vi "RT_DAQ Loop.vi"(8 "error in":errorcluster, 11 "Main Data":T1) -> (0 "error out":errorcluster)   [LabVIEW 2018]
uses:
  Data Def/RT_Main Data.ctl
  Data Def/RT_FPGA VI Reference.ctl
  Data Def/RT_Request Data.ctl
  <vilib>/Platform/TimedLoop/XDataNode/timing_clust.ctl
  <vilib>/Platform/TimedLoop/XDataNode/nitl_modes.ctl
  <vilib>/Platform/TimedLoop/XDataNode/wakeup.ctl
  Data Def/RT_Normal FGV Method.ctl
  <vilib>/Analysis/baseanly.llb/Mean (DBL).vi
  <vilib>/Utility/error.llb/Error Cluster From Error Code.vi
  <vilib>/rvi/errors/niLvFpgaAdjustHostInterfaceError.vi
  <vilib>/platform/TimedLoop/XDataNode/XDataNode.xnode
  <vilib>/rvi/interface/nirviReadWriteControl/nirviReadWriteControl.xnode
  <vilib>/Platform/TimedLoop/XDataNode/XDNodeRunTimeDep.lvlib
  NiFpgaLv.dll
  <vilib>/rvi/interface/Simulation/niFpgaSimulationCallBeginRW.vi
  <vilib>/Analysis/NI_AALBase.lvlib
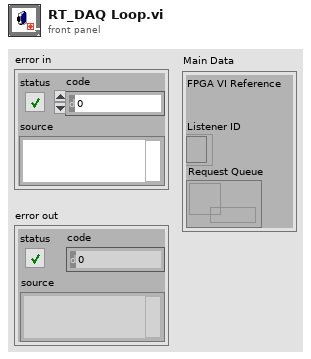
[diagram p1: front panel]
types:
  T1 = typedef "RT_Main Data.ctl" = cluster{"FPGA VI Reference":T2, "Listener ID":refnum<k5>, "Request Queue":refnum<queue>}
  T2 = typedef "RT_FPGA VI Reference.ctl" = refnum<k20>
  T3 = typedef "XDNodeRunTimeDep.lvlib/timing_clust.ctl" = cluster{"Expected End [f-1]":u64, "Actual End [f-1]":u64, "Finished Late? [f-1]":bool, "Expected End [i-1]":u64, "Actual End [i-1]":u64, "Finished Late? [i-1]":bool, "Expected Start [i]":u64, "Actual Start [i]":u64, "Expected Start [f]":u64, "Actual Start [f]":u64, "Source Name":string, "Structure Name":string, "Period":i64, "Deadline":i64, "Offset":i64, "Start":i64, "Priority":i32, "Timeout":i32, "Mode":T4, "Wakeup Reason":T5, "Error":errorcluster, "Source Type":string, "Secondary Source Type":string, "Global End Time":u64, "Global Start Time":u64, "Frame Duration":u64, "Iteration Duration":u64, "Assigned CPU":i32, "I/O Scan Engine Mode":u32}
  T4 = typedef "XDNodeRunTimeDep.lvlib/nitl_modes.ctl" = enum32{"No Change", "Process missed periods, maintain original phase", "Discard missed periods, maintain original phase", "Process missed periods, ignore original phase", "Discard missed periods, ignore original phase"}
  T5 = typedef "XDNodeRunTimeDep.lvlib/wakeup.ctl" = enum32{"Normal", "Aborted", "Asynchronous wakeup", "Timing source error", "Timed loop error", "Timeout"}
  T6 = typedef "RT_Normal FGV Method.ctl" = enum16{"Get", "Put"}
  T7 = typedef "RT_Configuration.ctl" = cluster{"Average Count":i32}
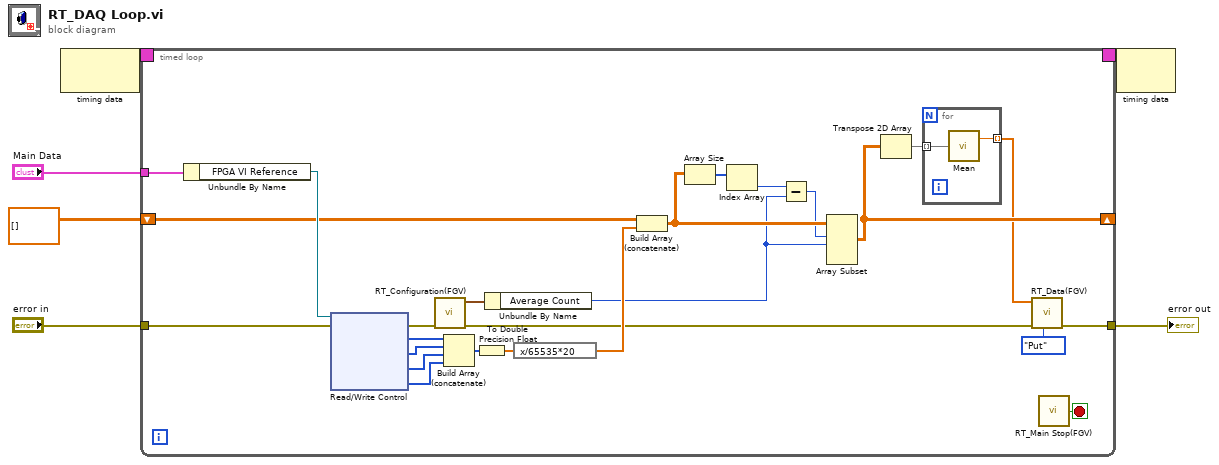
[diagram p0: block diagram]
diagram:
  n1 = node-c288() -> (w6:T3)  [unwired: 1 in]
  n2 = timed-loop {
    timing: w6 -> [_]
    timing-out: [_] -> w5
    tunnel: "error in" -> [w30]
    tunnel: "Main Data" -> [w31]
    shift-right: [w13] -> _
    shift-left: dbl[][] [] -> [w20]
    tunnel: [w8] -> w1
    stop <- w7 stop-if-true
    n3 = Unbundle By Name(w31) -> ("FPGA VI Reference"=w29:T2)
    n4 = xnode "Read/Write Control"("FPGA VI Reference In"=w29, "error in"=w30) -> ("error out"=w22:errorcluster, "C1 AI Data"=w27:i16[], "C2 AI Data"=w26:i16[], "C3 AI Data"=w25:i16[], "C4 AI Data"=w24:i16[])  [unwired: 1 out]
    n5 = call "RT_Configuration(FGV).vi"("error in"=w22) -> ("error out"=w11:errorcluster, "Configuration Out"=w21:T7)  [unwired: 9 in]
    n6 = Build Array (concatenate)(w27, w26, w25, w24) -> (w23:i16[])
    n7 = To Double Precision Float(number=w23) -> (double precision float=w28:dbl[])
    n8 = Unbundle By Name(w21) -> ("Average Count"=w14:i32)
    n9 = expression code="x/65535*20"(w28) -> (w19:dbl[])
    n10 = Build Array (concatenate)(w20, w19) -> (w18:dbl[][])
    n11 = Array Size(array=w18) -> (size(s)=w17:i32[])
    n12 = Index Array(array=w17) -> (element=w15:i32)  [unwired: 1 in]
    n13 = Subtract(x=w15, y=w14) -> (x-y=w16:i32)
    n14 = Array Subset(array=w18, index (row)=w16, length (row)=w14) -> (w13:dbl[][])  [unwired: 2 in]
    n15 = Transpose 2D Array(2D array=w13) -> (transposed array=w12:dbl[][])
    n16 = for {
      tunnel: w12 -> [w33] mode=indexing
      tunnel: [w32] -> w10 mode=indexing
      n17 = call-poly <vilib>:"Mean.vi"("X"=w33) -> ("mean"=w32:dbl)  [unwired: 1 out]
    }
    n18 = call "RT_Data(FGV).vi"("Normal FGV Method"=RT_Normal_FGV_Method."Put", "error in"=w11, "Data In"=w10) -> ("error out"=w8:errorcluster)  [unwired: 7 in, 1 out]
    n19 = call "RT_Main Stop(FGV).vi"() -> ("Stop Out"=w7:bool)  [unwired: 4 in]
  }
  "error out" <- w1
  n20 = node-c288(w5) -> ()  [unwired: 1 out]
